vi "Single Button Number.vi"(1 "Bool Array":bool[](array[boolean])) -> (0 "Number":i32)   [LabVIEW 2011]
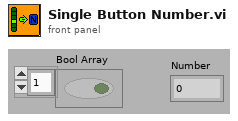
[diagram p1: front panel]
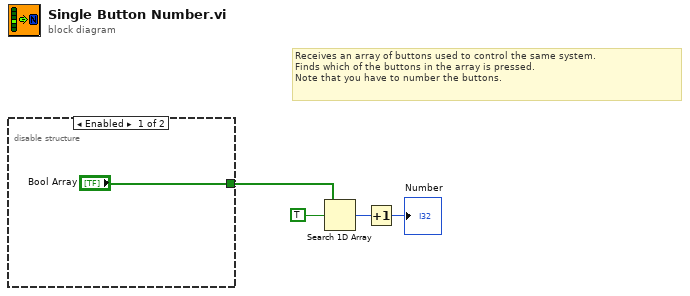
[diagram p0: block diagram]
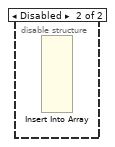
[diagram p2: hidden frame]
diagram:
  # "Receives an array of buttons used to control the same system.\nFinds which of the buttons in the array is pressed.\nNote that you have to number the buttons."
  n1 = disable-structure shown="Enabled" {
    disable-tunnel: ["Bool Array" _] -> w1
    frame Enabled {
    }
    frame Disabled {
      n2 = Insert Into Array() -> ()  [unwired: 8 in, 1 out]
    }
  }
  n3 = Search 1D Array(1D array=w1, element=TRUE) -> (index of element=w3:i32)  [unwired: 1 out]
  n4 = Increment(x=w3) -> (x+1=→"Number":i32)
